vi "LJLogUD read config.vi"(0 "Working Directory":path, 5 "filename":string="ljstreamud.cfg", 7 "ChP Default":string="0#!#1#!#2#!#3#!#4#!#5#!#6#!#7#!#8#!#9#!#10#!#11#!#12#!#13#!#14#!#15#!#") -> (1 "Data File Prefix":string="data", 2 "Scan Rate (Hz)":dbl=500.0 format="%.3f", 3 "Graph History":i32=1000 min=0, 4 "# Channels":i32=4, 6 "Disable Scaling":bool, 8 "Max File Size (Bytes)":i32=1048576, 9 "Write To File":bool, 10 "Channel Setup":T1={"+Ch"=["0", "1", "2", "3", "4", "5", "6", "7"], "-Ch"=["199", "199", "199", "199", "199", "199", "199", "199"], "Ranges"=[0, 0, 0, 0, 0, 0, 0, 0], "Scaling Equation"=["y=v0", "y=v1", "y=v2", "y=v3", "y=v4", "y=v5", "y=v6", "y=v7"], "Graph?"=[]} {"Ranges" items=["LJ_rgBIP10V", "LJ_rgBIP5V", "LJ_rgUNI5V", "LJ_rgUNI2P5V", "LJ_rgUNI1P25V", "LJ_rgBIP1V", "LJ_rgUNIP625V", "LJ_rgBIPP1V", "LJ_rgBIPP01V"]}, 11 "Good Config File":bool, 12 "Interval (ms)":u32=500, 13 "Resolution":u8, 14 "SettlingFactor":u8, 15 "error out":errorcluster)   [LabVIEW 2020]
uses:
  <vilib>/Utility/config.llb/Read Key (String).vi
  <vilib>/Utility/config.llb/Read Key (U32).vi
  <vilib>/Utility/config.llb/Read Key (Double).vi
  <vilib>/Utility/config.llb/Read Key (I32).vi
  <vilib>/Utility/config.llb/Read Key (Boolean).vi
  <vilib>/Utility/config.llb/NI_LVConfig.lvlib
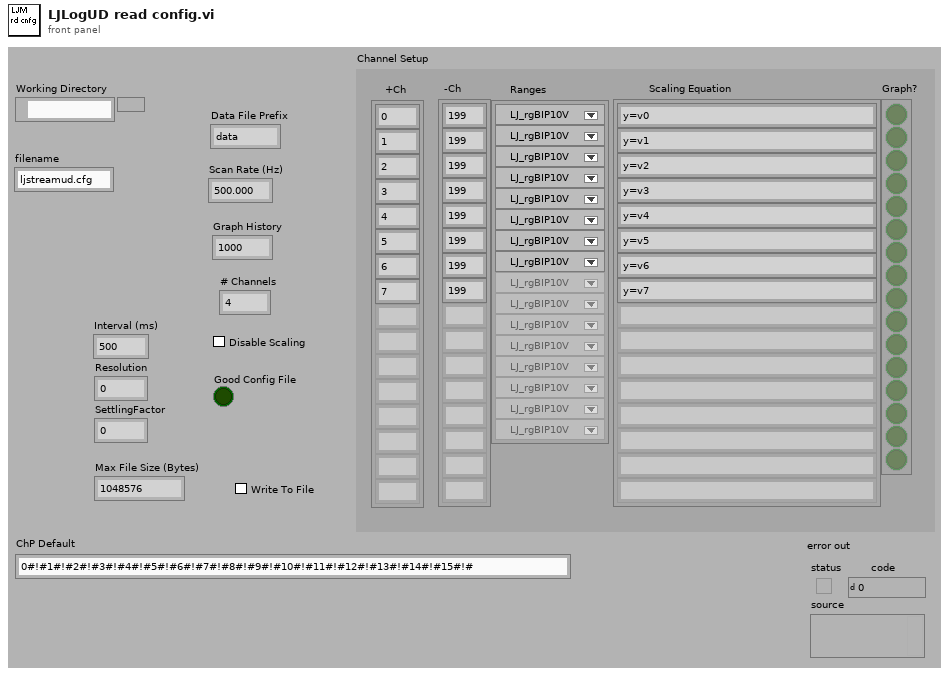
[diagram p1: front panel]
types:
  T1 = cluster{"+Ch":string[], "-Ch":string[], "Ranges":u16[], "Scaling Equation":string[], "Graph?":bool[]}
  T2 = typedef "NI_LVConfig.lvlib/Config Data RefNum.ctl" = refnum<k1>
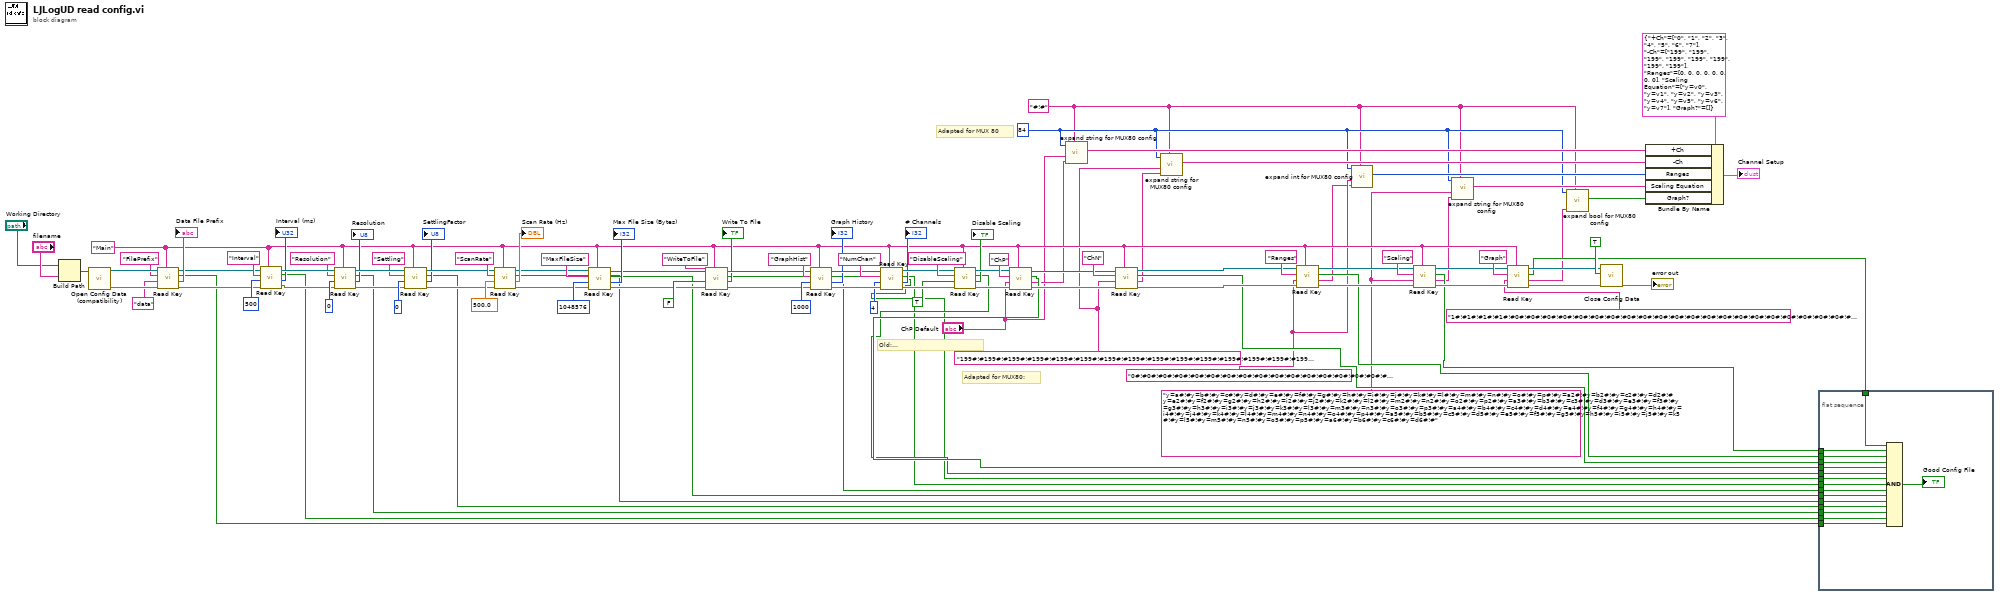
[diagram p0: block diagram]
diagram:
  w7 = "y=a#!#y=b#!#y=c#!#y=d#!#y=e#!#y=f#!#y=g#!#y=h#!#y=i#!#y=j#!#y=k#!#y=l#!#y=m#!#y=n#!#y=o#!#y=p#!#y=a2#!#y=b2#!#y=c2#!#y=d2#!#y=e2#!#y=f2#!#y=g2#!#y=h2#!#y=i2#!#y=j2#!#y=k2#!#y=l2#!#y=m2#!#y=n2#!#y=o2#!#y=p2#!#y=a3#!#y=b3#!#y=c3#!#y=d3#!#y=e3#!#y=f3#!#y=g3#!#y=h3#!#y=i3#!#y=j3#!#y=k3#!#y=l3#!#y=m3#!#y=n3#!#y=o3#!#y=p3#!#y=a4#!#y=b4#!#y=c4#!#y=d4#!#y=e4#!#y=f4#!#y=g4#!#y=h4#!#y=i4#!#y=j4#!#y=k4#!#y=l4#!#y=m4#!#y=n4#!#y=o4#!#y=p4#!#y=a5#!#y=b5#!#y=c5#!#y=d5#!#y=e5#!#y=f5#!#y=g5#!#y=h5#!#y=i5#!#y=j5#!#y=k5#!#y=l5#!#y=m5#!#y=n5#!#y=o5#!#y=p5#!#y=a6#!#y=b6#!#y=c6#!#y=d6#!#" ("Data File Prefix")
  w10 = "0#!#0#!#0#!#0#!#0#!#0#!#0#!#0#!#0#!#0#!#0#!#0#!#0#!#0#!#0#!#0#!#0#!#0#!#0#!#0#!#0#!#0#!#0#!#0#!#0#!#0#!#0#!#0#!#0#!#0#!#0#!#0#!#0#!#0#!#0#!#0#!#0#!#0#!#0#!#0#!#0#!#0#!#0#!#0#!#0#!#0#!#0#!#0#!#0#!#0#!#0#!#0#!#0#!#0#!#0#!#0#!#0#!#0#!#0#!#0#!#0#!#0#!#0#!#0#!#0#!#0#!#0#!#0#!#0#!#0#!#0#!#0#!#0#!#0#!#0#!#0#!#0#!#0#!#0#!#0#!#0#!#0#!#0#!#0#!#" ("Data File Prefix")
  w15 = "199#!#199#!#199#!#199#!#199#!#199#!#199#!#199#!#199#!#199#!#199#!#199#!#199#!#199#!#199#!#199#!#199#!#199#!#199#!#199#!#199#!#199#!#199#!#199#!#199#!#199#!#199#!#199#!#199#!#199#!#199#!#199#!#199#!#199#!#199#!#199#!#199#!#199#!#199#!#199#!#199#!#199#!#199#!#199#!#199#!#199#!#199#!#199#!#199#!#199#!#199#!#199#!#199#!#199#!#199#!#199#!#199#!#199#!#199#!#199#!#199#!#199#!#199#!#199#!#199#!#199#!#199#!#199#!#199#!#199#!#199#!#199#!#199#!#199#!#199#!#199#!#199#!#199#!#199#!#199#!#199#!#199#!#199#!#199#!#" ("Data File Prefix")
  w2 = 84
  w1 = "#!#" ("delimiter (Tab)")
  w33 = "Main" ("section")
  # "Adapted for MUX 80"
  # "Adapted for MUX80:"
  # "Old: 199#!#199#!#199#!#199#!#199#!#199#!#199#!#199#!#199#!#199#!#199#!#199#!#199#!#199#!#199#!#199#!#"
  n1 = Build Path(base path="Working Directory", name or relative path="filename") -> (appended path=w106:path)
  n2 = call <vilib>:"Open Config Data (compatibility).vi"("configuration file path"=w106) -> ("error out"=w103:errorcluster, "refnum"=w104:T2)  [unwired: 8 in, 1 out]
  n3 = call-poly <vilib>:"Read Key.vi"("section"=w33, "error in (no error)"=w103, "default value"="data" ("Data File Prefix"), "key"="FilePrefix", "refnum"=w104) -> ("error out"=w53:errorcluster, "value"=→"Data File Prefix":string, "found?"=w18:bool, "refnum out"=w51:T2)  [unwired: 3 in]
  n4 = call-poly <vilib>:"Read Key.vi"("section"=w33, "error in (no error)"=w53, "default value"=u32 500 ("Scan Rate (Hz)"), "key"="Interval", "refnum"=w51) -> ("error out"=w58:errorcluster, "value"=→"Interval (ms)":u32, "found?"=w19:bool, "refnum out"=w57:T2)  [unwired: 3 in]
  n5 = call-poly <vilib>:"Read Key.vi"("section"=w33, "error in (no error)"=w58, "default value"=u8 0 ("Graph History"), "key"="Resolution", "refnum"=w57) -> ("error out"=w60:errorcluster, "value"=→"Resolution":u32, "found?"=w20:bool, "refnum out"=w59:T2)  [unwired: 3 in]
  n6 = call-poly <vilib>:"Read Key.vi"("section"=w33, "error in (no error)"=w60, "default value"=u8 0 ("# Channels"), "key"="Settling", "refnum"=w59) -> ("error out"=w52:errorcluster, "value"=→"SettlingFactor":u32, "found?"=w21:bool, "refnum out"=w50:T2)  [unwired: 3 in]
  n7 = call-poly <vilib>:"Read Key.vi"("section"=w33, "error in (no error)"=w52, "default value"=500.0 ("Scan Rate (Hz)"), "key"="ScanRate", "refnum"=w50) -> ("error out"=w43:errorcluster, "value"=→"Scan Rate (Hz)":dbl, "found?"=w22:bool, "refnum out"=w42:T2)  [unwired: 3 in]
  n8 = call-poly <vilib>:"Read Key.vi"("section"=w33, "error in (no error)"=w43, "default value"=1048576 ("Graph History"), "key"="MaxFileSize", "refnum"=w42) -> ("error out"=w37:errorcluster, "value"=→"Max File Size (Bytes)":i32, "found?"=w23:bool, "refnum out"=w38:T2)  [unwired: 3 in]
  n9 = call-poly <vilib>:"Read Key.vi"("section"=w33, "error in (no error)"=w37, "default value"=FALSE, "key"="WriteToFile", "refnum"=w38) -> ("error out"=w35:errorcluster, "value"=→"Write To File":bool, "found?"=w24:bool, "refnum out"=w36:T2)  [unwired: 3 in]
  n10 = call-poly <vilib>:"Read Key.vi"("section"=w33, "error in (no error)"=w35, "default value"=1000 ("Graph History"), "key"="GraphHist", "refnum"=w36) -> ("error out"=w98:errorcluster, "value"=→"Graph History":i32, "found?"=w25:bool, "refnum out"=w99:T2)  [unwired: 3 in]
  n11 = call-poly <vilib>:"Read Key.vi"("section"=w33, "error in (no error)"=w98, "default value"=4 ("# Channels"), "key"="NumChan", "refnum"=w99) -> ("error out"=w80:errorcluster, "value"=→"# Channels":i32, "found?"=w26:bool, "refnum out"=w81:T2)  [unwired: 3 in]
  n12 = call-poly <vilib>:"Read Key.vi"("section"=w33, "error in (no error)"=w80, "default value"=TRUE, "key"="DisableScaling", "refnum"=w81) -> ("error out"=w78:errorcluster, "value"=→"Disable Scaling":bool, "found?"=w27:bool, "refnum out"=w77:T2)  [unwired: 3 in]
  n13 = call-poly <vilib>:"Read Key.vi"("section"=w33, "error in (no error)"=w78, "default value"="ChP Default", "key"="ChP", "refnum"=w77) -> ("error out"=w93:errorcluster, "value"=w17:string, "found?"=w28:bool, "refnum out"=w94:T2)  [unwired: 3 in]
  n14 = call "expand string for MUX80 config.vi"("RegEx"=w1, "Input Config Str"=w17, "Default Config Str"="ChP Default", "NumChannels"=w2) -> ("Output Config Arr"=w13:string[])  [unwired: 6 in, 1 out]
  n15 = call-poly <vilib>:"Read Key.vi"("section"=w33, "error in (no error)"=w93, "default value"=w15, "key"="ChN", "refnum"=w94) -> ("error out"=w92:errorcluster, "value"=w14:string, "found?"=w29:bool, "refnum out"=w91:T2)  [unwired: 3 in]
  n16 = call "expand string for MUX80 config.vi"("RegEx"=w1, "Input Config Str"=w14, "Default Config Str"=w15, "NumChannels"=w2) -> ("Output Config Arr"=w12:string[])  [unwired: 6 in, 1 out]
  n17 = call-poly <vilib>:"Read Key.vi"("section"=w33, "error in (no error)"=w92, "default value"=w10, "key"="Ranges", "refnum"=w91) -> ("error out"=w89:errorcluster, "value"=w9:string, "found?"=w30:bool, "refnum out"=w88:T2)  [unwired: 3 in]
  n18 = call "expand int for MUX80 config.vi"("RegEx"=w1, "Input Config Str"=w9, "Default Config Str"=w10, "NumChannels"=w2) -> ("Output Config Arr"=w11:i32[])  [unwired: 6 in, 1 out]
  n19 = call-poly <vilib>:"Read Key.vi"("section"=w33, "error in (no error)"=w89, "default value"=w7, "key"="Scaling", "refnum"=w88) -> ("error out"=w75:errorcluster, "value"=w6:string, "found?"=w31:bool, "refnum out"=w72:T2)  [unwired: 3 in]
  n20 = call "expand string for MUX80 config.vi"("RegEx"=w1, "Input Config Str"=w6, "Default Config Str"=w7, "NumChannels"=w2) -> ("Output Config Arr"=w8:string[])  [unwired: 6 in, 1 out]
  n21 = call-poly <vilib>:"Read Key.vi"("section"=w33, "error in (no error)"=w75, "default value"="1#!#1#!#1#!#1#!#0#!#0#!#0#!#0#!#0#!#0#!#0#!#0#!#0#!#0#!#0#!#0#!#0#!#0#!#0#!#0#!#0#!#0#!#0#!#0#!#0#!#0#!#0#!#0#!#0#!#0#!#0#!#0#!#0#!#0#!#0#!#0#!#0#!#0#!#0#!#0#!#0#!#0#!#0#!#0#!#0#!#0#!#0#!#0#!#0#!#0#!#0#!#0#!#0#!#0#!#0#!#0#!#0#!#0#!#0#!#0#!#0#!#0#!#0#!#0#!#0#!#0#!#0#!#0#!#0#!#0#!#0#!#0#!#0#!#0#!#0#!#0#!#0#!#0#!#0#!#0#!#0#!#0#!#0#!#0#!#" ("Data File Prefix"), "key"="Graph", "refnum"=w72) -> ("error out"=w74:errorcluster, "value"=w4:string, "found?"=w32:bool, "refnum out"=w73:T2)  [unwired: 3 in]
  n22 = call "expand bool for MUX80 config.vi"("RegEx"=w1, "Input Config Str"=w4, "NumChannels"=w2) -> ("Output Config Arr"=w5:bool[])  [unwired: 8 in]
  n23 = call <vilib>:"Close Config Data.vi"("error in (no error)"=w74, "write file if changed (T)"=TRUE ("write configuration file? (F)"), "refnum"=w73) -> ("error out"=→"error out":errorcluster)  [unwired: 7 in, 1 out]
  n24 = Bundle By Name(cluster=T1 {"+Ch"=["0", "1", "2", "3", "4", "5", "6", "7"], "-Ch"=["199", "199", "199", "199", "199", "199", "199", "199"], "Ranges"=[0, 0, 0, 0, 0, 0, 0, 0], "Scaling Equation"=["y=v0", "y=v1", "y=v2", "y=v3", "y=v4", "y=v5", "y=v6", "y=v7"], "Graph?"=[]} ("Channel Setup"), "+Ch"=w13, "-Ch"=w12, "Ranges"=w11, "Scaling Equation"=w8, "Graph?"=w5) -> (→"Channel Setup":T1)
  n25 = flat-sequence {
    tunnel: w32 -> [w123]
    tunnel: w31 -> [w122]
    tunnel: w30 -> [w121]
    tunnel: w29 -> [w120]
    tunnel: w28 -> [w119]
    tunnel: w27 -> [w118]
    tunnel: w26 -> [w117]
    tunnel: w25 -> [w116]
    tunnel: w24 -> [w115]
    tunnel: w23 -> [w114]
    tunnel: w22 -> [w113]
    tunnel: w21 -> [w112]
    tunnel: w20 -> [w111]
    tunnel: w19 -> [w110]
    tunnel: w18 -> [w109]
    frame #0 {
      n26 = Compound Arithmetic op=AND(w123, w122, w121, w120, w119, w118, w117, w116, w115, w114, w113, w112, w111, w110, w109) -> (→"Good Config File":bool)
    }
  }
